vi "Tree_FocusPath_Tests.vi"(11 "error in":errorcluster) -> (15 "error out":errorcluster)   [LabVIEW 2016, in "DronaTest.lvlib"]
uses:
  DronaTest.lvlib
  APIs/Stimulus/ControlValue/SetValueAuto.vi
  APIs/Stimulus/ControlValue/Controls/Tree/SetValueByHierarchicalPath.vi
  APIs/Assert/AssertControlValue/Controls/Tree/AssertValueByFocusNamePath.vi
  <vilib>/addons/_JKI Toolkits/Caraya/classes/Assert/Assert Error.vi
  <vilib>/addons/_JKI Toolkits/Caraya/classes/Assert/Assert Equal Value_Variant.vi
  <vilib>/addons/_JKI Toolkits/Caraya/classes/Test/Test.lvclass
  Drona.lvlib
  <vilib>/SLL Toolkit/SLL Debug/SLL Debug.lvlib
  APIs/Stimulus/ControlValue/ControlValue.lvlib
  <vilib>/addons/_JKI Toolkits/Caraya/classes/Assert/Assert.lvclass
  APIs/Stimulus/ControlValue/Controls/Tree/StimulusTree.lvlib
  APIs/Assert/AssertControlValue/Controls/Tree/AssertTree.lvlib
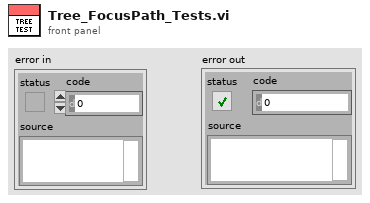
[diagram p1: front panel]
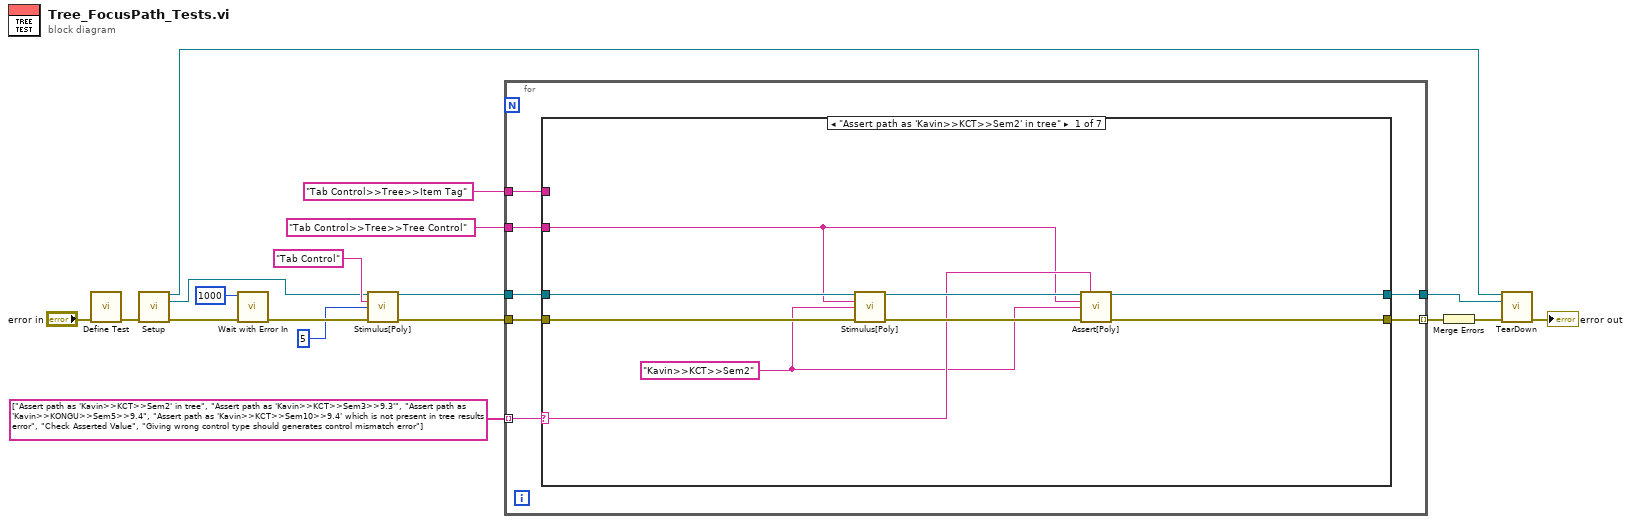
[diagram p0: block diagram]
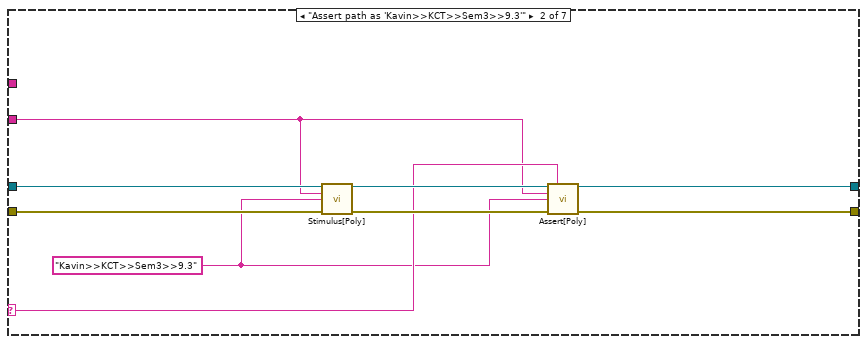
[diagram p2: hidden frame]
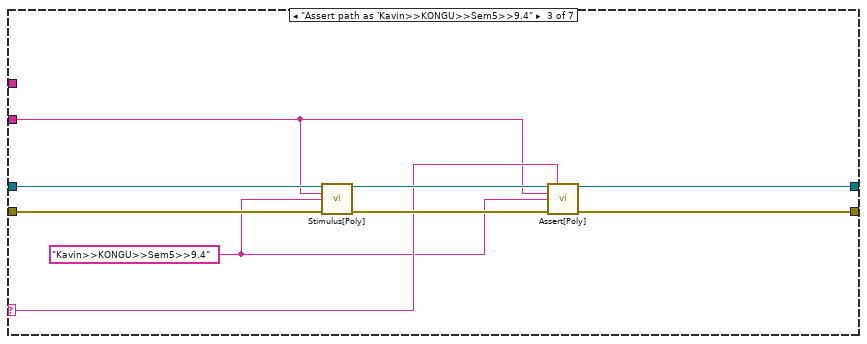
[diagram p3: hidden frame]
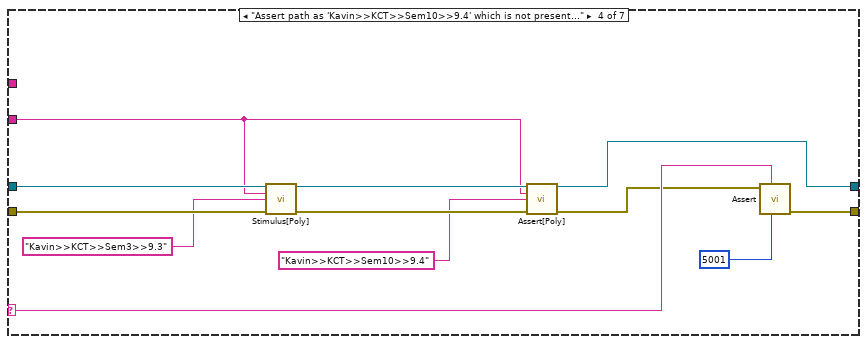
[diagram p4: hidden frame]
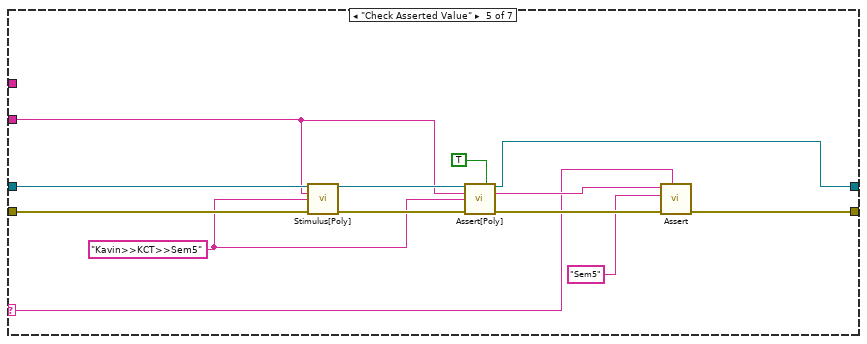
[diagram p5: hidden frame]
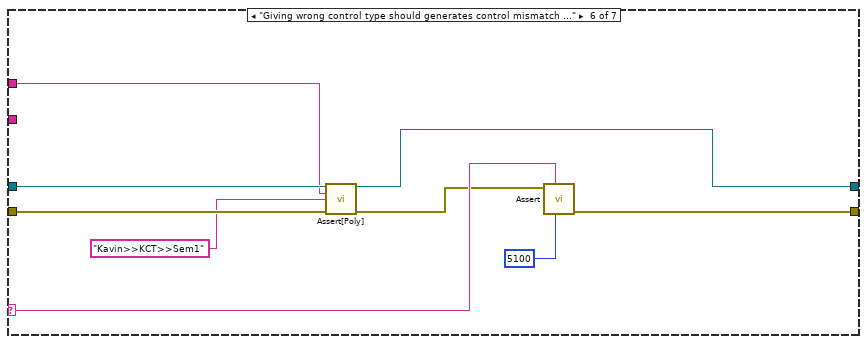
[diagram p6: hidden frame]
diagram:
  n1 = call <vilib>:"Define Test.vi"("error in (no error)"="error in") -> ("error out"=w7:errorcluster)  [unwired: 9 in, 1 out]
  n2 = call "Setup.vi"("error in (no error)"=w7) -> ("Application Ref"=w2:refnum<vi>, "VI out"=w6:refnum<vi>, "error out"=w5:errorcluster)  [unwired: 12 in]
  n3 = call <vilib>:"Wait with Error In.vi"("error in (no error)"=w5, "milliseconds to wait"=u32 1000) -> ("error out"=w16:errorcluster)  [unwired: 9 in]
  n4 = call-poly "Stimulus[Poly].vi"("VI Reference In"=w6, "Control Path"="Tab Control", "Value (Signaling)"=5, "error in"=w16) -> ("VI Reference Out"=w12:refnum<vi>, "error out"=w15:errorcluster)  [unwired: 10 in]
  n5 = for {
    tunnel: w12 -> [w24]
    tunnel: "Tab Control>>Tree>>Tree Control" ("Control Path") -> [w23]
    tunnel: "Tab Control>>Tree>>Item Tag" ("Control Path") -> [w22]
    tunnel: string[] ["Assert path as 'Kavin>>KCT>>Sem2' in tree", "Assert path as 'Kavin>>KCT>>Sem3>>9.3'", "Assert path as 'Kavin>>KONGU>>Sem5>>9.4", "Assert path as 'Kavin>>KCT>>Sem10>>9.4' which is not present in tree results error", "Check Asserted Value", "Giving wrong control type should generates control mismatch error"] -> [w20] mode=indexing
    tunnel: [w19] -> w3
    tunnel: w15 -> [w25]
    tunnel: [w21] -> w8 mode=indexing
    n6 = case shown="\"Assert path as 'Kavin>>KCT>>Sem2' in tree\"" w20 {
      selector: w20 -> [w28 w37 w46 w60 w68 w85 _]
      tunnel: w25 -> [w34 w43 w52 w64 w76 w83 w88]
      tunnel: w24 -> [w33 w42 w51 w63 w74 w81 w87]
      tunnel: w23 -> [w26 w35 w44 w54 w66 _ _]
      tunnel: w22 -> [_ _ _ _ _ w80 _]
      tunnel: [w30 w39 w48 w62 w67 w86 w88] -> w21
      tunnel: [w29 w38 w47 w55 w77 w78 w87] -> w19
      frame "Assert path as 'Kavin>>KCT>>Sem2' in tree" {
        w27 = "Kavin>>KCT>>Sem2" ("Item Name")
        n7 = call-poly "Stimulus[Poly].vi"("VI Reference In"=w33, "Control Path"=w26, "Hierarchical Path"=w27, "Error In"=w34) -> ("VI Reference Out"=w31:refnum<vi>, "Error Out"=w32:errorcluster)  [unwired: 10 in]
        n8 = call-poly "Assert[Poly].vi"("VI Reference In"=w31, "Test Label"=w28, "Control Path"=w26, "Focus Item Path"=w27, "Error In"=w32) -> ("VI Reference Out"=w29:refnum<vi>, "Error Out"=w30:errorcluster)  [unwired: 8 in, 1 out]
      }
      frame "Assert path as 'Kavin>>KCT>>Sem3>>9.3'" {
        w36 = "Kavin>>KCT>>Sem3>>9.3" ("Item Name")
        n9 = call-poly "Stimulus[Poly].vi"("VI Reference In"=w42, "Control Path"=w35, "Hierarchical Path"=w36, "Error In"=w43) -> ("VI Reference Out"=w40:refnum<vi>, "Error Out"=w41:errorcluster)  [unwired: 10 in]
        n10 = call-poly "Assert[Poly].vi"("VI Reference In"=w40, "Test Label"=w37, "Control Path"=w35, "Focus Item Path"=w36, "Error In"=w41) -> ("VI Reference Out"=w38:refnum<vi>, "Error Out"=w39:errorcluster)  [unwired: 8 in, 1 out]
      }
      frame "Assert path as 'Kavin>>KONGU>>Sem5>>9.4" {
        w45 = "Kavin>>KONGU>>Sem5>>9.4" ("Item Name")
        n11 = call-poly "Stimulus[Poly].vi"("VI Reference In"=w51, "Control Path"=w44, "Hierarchical Path"=w45, "Error In"=w52) -> ("VI Reference Out"=w49:refnum<vi>, "Error Out"=w50:errorcluster)  [unwired: 10 in]
        n12 = call-poly "Assert[Poly].vi"("VI Reference In"=w49, "Test Label"=w46, "Control Path"=w44, "Focus Item Path"=w45, "Error In"=w50) -> ("VI Reference Out"=w47:refnum<vi>, "Error Out"=w48:errorcluster)  [unwired: 8 in, 1 out]
      }
      frame "Assert path as 'Kavin>>KCT>>Sem10>>9.4' which is not present in tree results error" {
        n13 = call-poly "Stimulus[Poly].vi"("VI Reference In"=w63, "Control Path"=w54, "Hierarchical Path"="Kavin>>KCT>>Sem3>>9.3" ("Item Name"), "Error In"=w64) -> ("VI Reference Out"=w56:refnum<vi>, "Error Out"=w58:errorcluster)  [unwired: 10 in]
        n14 = call-poly "Assert[Poly].vi"("VI Reference In"=w56, "Control Path"=w54, "Focus Item Path"="Kavin>>KCT>>Sem10>>9.4" ("Item Name"), "Error In"=w58) -> ("VI Reference Out"=w55:refnum<vi>, "Error Out"=w57:errorcluster)  [unwired: 9 in, 1 out]
        n15 = call-poly <vilib>:"Assert.vi"("error code (1)"=5001, "Label"=w60, "Error?"=w57) -> ("error out"=w62:errorcluster)  [unwired: 7 in, 1 out]
      }
      frame "Check Asserted Value" {
        w72 = "Kavin>>KCT>>Sem5" ("Item Name")
        n16 = call-poly "Stimulus[Poly].vi"("VI Reference In"=w74, "Control Path"=w66, "Hierarchical Path"=w72, "Error In"=w76) -> ("VI Reference Out"=w73:refnum<vi>, "Error Out"=w75:errorcluster)  [unwired: 10 in]
        n17 = call-poly "Assert[Poly].vi"("VI Reference In"=w73, "Assert Only? (F)"=TRUE, "Control Path"=w66, "Focus Item Path"=w72, "Error In"=w75) -> ("VI Reference Out"=w77:refnum<vi>, "Asserted Value"=w70:string, "Error Out"=w71:errorcluster)  [unwired: 8 in]
        n18 = call-poly <vilib>:"Assert.vi"("Label"=w68, "error in (no error)"=w71, "Y"="Sem5" ("Asserted Value"), "X"=w70) -> ("error out"=w67:errorcluster)  [unwired: 6 in, 1 out]
      }
      frame "Giving wrong control type should generates control mismatch error" {
        n19 = call-poly "Assert[Poly].vi"("VI Reference In"=w81, "Control Path"=w80, "Focus Item Path"="Kavin>>KCT>>Sem1" ("Item Name"), "Error In"=w83) -> ("VI Reference Out"=w78:refnum<vi>, "Error Out"=w82:errorcluster)  [unwired: 9 in, 1 out]
        n20 = call-poly <vilib>:"Assert.vi"("error code (1)"=5100, "Label"=w85, "Error?"=w82) -> ("error out"=w86:errorcluster)  [unwired: 7 in, 1 out]
      }
      frame Default {
      }
    }
  }
  n21 = Merge Errors(w8) -> (w4:errorcluster)
  n22 = call "TearDown.vi"("Application Ref"=w2, "VI in"=w3, "error in (no error)"=w4) -> ("error out"=→"error out":errorcluster)  [unwired: 12 in]
